vi "PolarToRect.vi"(10 "theta":dbl[](array[numeric]), 11 "r":dbl[](array[numeric])) -> (3 "Rectangular Coordinates":cluster{dbl[], dbl[]})   [LabVIEW 2020]
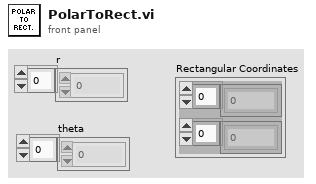
[diagram p1: front panel]
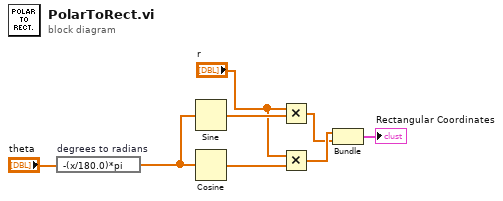
[diagram p0: block diagram]
diagram:
  n1 = expression code="-(x/180.0)*pi" "degrees to radians"("theta") -> (w3:dbl[])
  n2 = Sine(x=w3) -> (sin(x)=w8:dbl[])
  n3 = Cosine(x=w3) -> (cos(x)=w6:dbl[])
  n4 = Multiply(x="r", y=w8) -> (x*y=w1:dbl[])
  n5 = Multiply(x="r", y=w6) -> (x*y=w2:dbl[])
  n6 = Bundle(w2, w1) -> (→"Rectangular Coordinates":cluster{dbl[], dbl[]})  [unwired: 1 in]
